vi "Copy Sign Double Array.vi"(1 "y":dbl, 2 "x":dbl[](array[numeric])) -> (0 "x out":dbl[](array[numeric]))   [LabVIEW 2025]
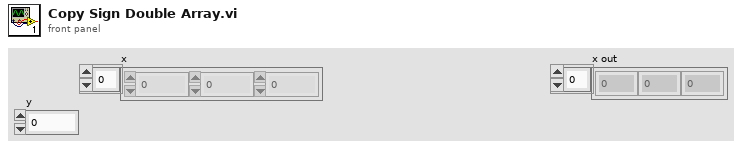
[diagram p1: front panel]
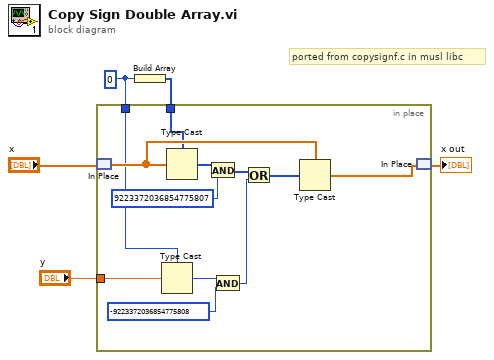
[diagram p0: block diagram]
diagram:
  w1 = i64 0
  # "ported from copysignf.c in musl libc"
  n1 = Build Array(w1) -> (w2:i64[])
  n2 = in-place {
    in-place-border: "y" -> [w14]
    in-place-border: w2 -> [w7]
    in-place-border: w1 -> [w6]
    n3 = in-place-match #1("x") -> (w9:dbl[])
    n4 = Type Cast(type=w6, x=w14) -> (*(type *) &x=w13:i64)
    n5 = Type Cast(type=w7, x=w9) -> (*(type *) &x=w17:i64[])
    n6 = And(x=w17, y=i64 9223372036854775807) -> (x .and. y?=w15:i64[])
    n7 = And(x=w13, y=i64 -9223372036854775808) -> (x .and. y?=w11:i64)
    n8 = Or(x=w15, y=w11) -> (x .or. y?=w10:i64[])
    n9 = Type Cast(type=w9, x=w10) -> (*(type *) &x=w8:dbl[])
    n10 = in-place-match #1(w8) -> (→"x out":dbl[])
  }
